vi "Problem1.8-GenerateUniformDeviates-SubVI.vi"() -> (2 "number: 0 to 1":dbl, 3 "Numeric":dbl)   [LabVIEW 2019]
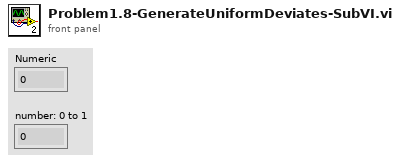
[diagram p1: front panel]
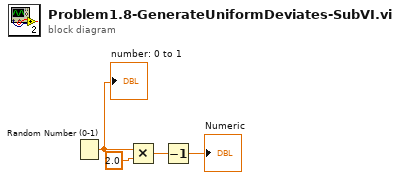
[diagram p0: block diagram]
diagram:
  n1 = Random Number (0-1)() -> (number: 0 to 1=w1:dbl)
  "number: 0 to 1" <- w1
  n2 = Multiply(x=w1, y=2.0) -> (x*y=w3:dbl)
  n3 = Decrement(x=w3) -> (x-1=→"Numeric":dbl)
